vi "Set Rate (Percent).vi"(8 "error in (no error)":errorcluster, 10 "Rate (Percentage)":dbl, 11 "Motors with Encoders in":refnum<class "Motors with Encoders.lvclass">) -> (0 "error out":errorcluster, 3 "Motors with Encoders out":refnum<class "Motors with Encoders.lvclass">)   [LabVIEW 2014, in "Motors with Encoders.lvlib" / "Motors with Encoders.lvclass"]
uses:
  Motors with Encoders.lvclass
  Motors with Encoders.lvclass/Motors with Encoders.ctl
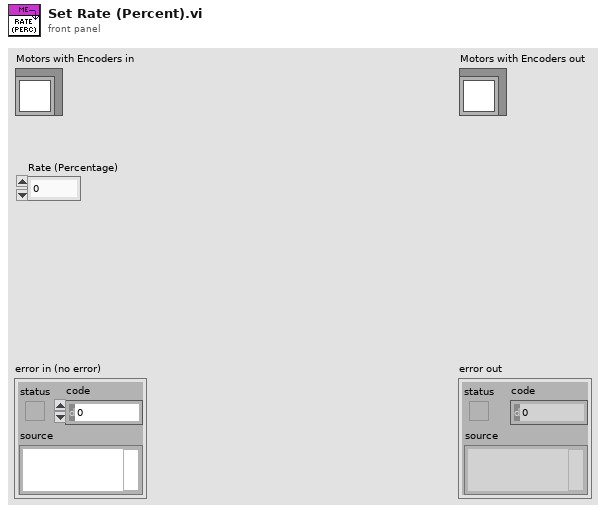
[diagram p1: front panel]
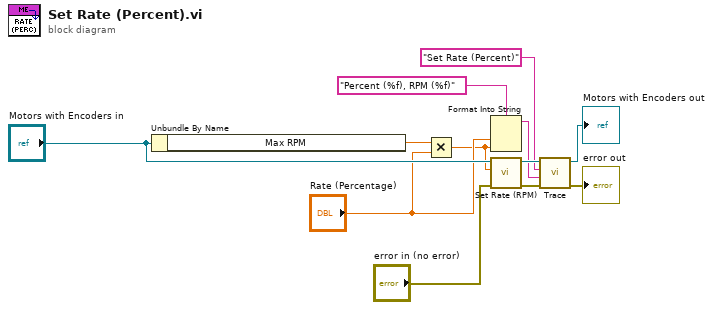
[diagram p0: block diagram]
diagram:
  n1 = Unbundle By Name("Motors with Encoders in") -> ("Max RPM"=w12:dbl)
  n2 = Multiply(x=w12, y="Rate (Percentage)") -> (x*y=w1:dbl)
  n3 = Format Into String(format string="Percent (%f), RPM (%f)", "Rate (Percentage)", w1) -> (resulting string=w3:string)  [unwired: 2 in, 1 out]
  n4 = call-dynamic "Set Rate (RPM).vi"("error in (no error)"="error in (no error)", "Rate (RPM)"=w1, "Motors with Encoders in"="Motors with Encoders in") -> ("error out"=w7:errorcluster, "Motors with Encoders out"=w10:refnum<class "Motors with Encoders.lvclass">)  [unwired: 7 in]
  n5 = call-dynamic "Trace.vi"("error in (no error)"=w7, "System Message"=w3, "System Action"="Set Rate (Percent)", "System Actor in"=w10) -> ("error out"=→"error out":errorcluster, "System Actor out"=→"Motors with Encoders out":refnum<class "Motors with Encoders.lvclass">)  [unwired: 6 in]
